vi "remove PID from array.vi"(8 "error in":errorcluster, 10 "line number":i32, 11 "operations table":T1) -> (0 "error out":errorcluster)   [LabVIEW 2014, in "Tagbus PID Module editor node.lvclass"]
uses:
  Tagbus PID Module editor node.lvclass
  PID array reference.ctl
  PID array element.ctl
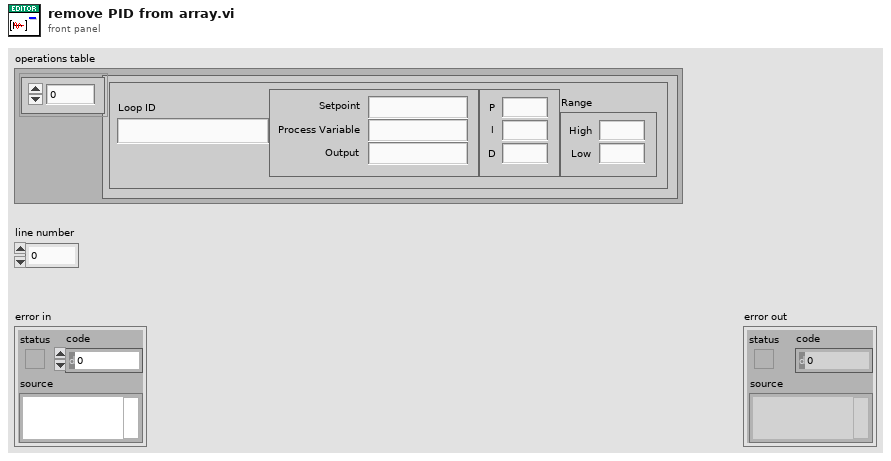
[diagram p1: front panel]
types:
  T1 = typedef "Tagbus PID Module editor node.lvclass/PID array reference.ctl" = refnum<vi>
  T2 = typedef "Tagbus PID Module editor node.lvclass/PID array element.ctl" = cluster{"Loop ID":string, "Tags":cluster{"Setpoint":string, "Process Variable":string, "Output":string}, "Gains":cluster{"P":dbl, "I":dbl, "D":dbl}, "Range":cluster{"High":dbl, "Low":dbl}}
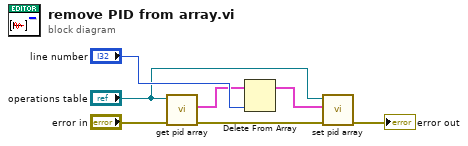
[diagram p0: block diagram]
diagram:
  n1 = call "get pid array.vi"("error in (no error)"="error in", "Array in"="operations table") -> ("error out"=w2:errorcluster, "Value"=w5:T2[])  [unwired: 7 in, 1 out]
  n2 = Delete From Array(array=w5, index="line number") -> (array with subset deleted=w4:T2[])  [unwired: 1 in, 1 out]
  n3 = call "set pid array.vi"("error in (no error)"=w2, "Array"=w4, "Array in"="operations table") -> ("error out"=→"error out":errorcluster)  [unwired: 7 in, 1 out]
